vi "SWERVE_DRIVE_DASH_WRITE.vi"   [LabVIEW 2023]
uses:
  SWERVE_DRIVE_GLOBALS.vi
  <vilib>/Rock Robotics/Network Tables/NT Write Numeric Array.vi
  <vilib>/Rock Robotics/Network Tables/NT Write Boolean Array.vi
  <vilib>/Rock Robotics/Network Tables/NT Write Boolean.vi
  <vilib>/Rock Robotics/Network Tables/NT Write Number.vi
  <vilib>/Rock Robotics/WPI/ThirdParty/JAS_Junk/TrajLib/Trajectory_Library.lvlib
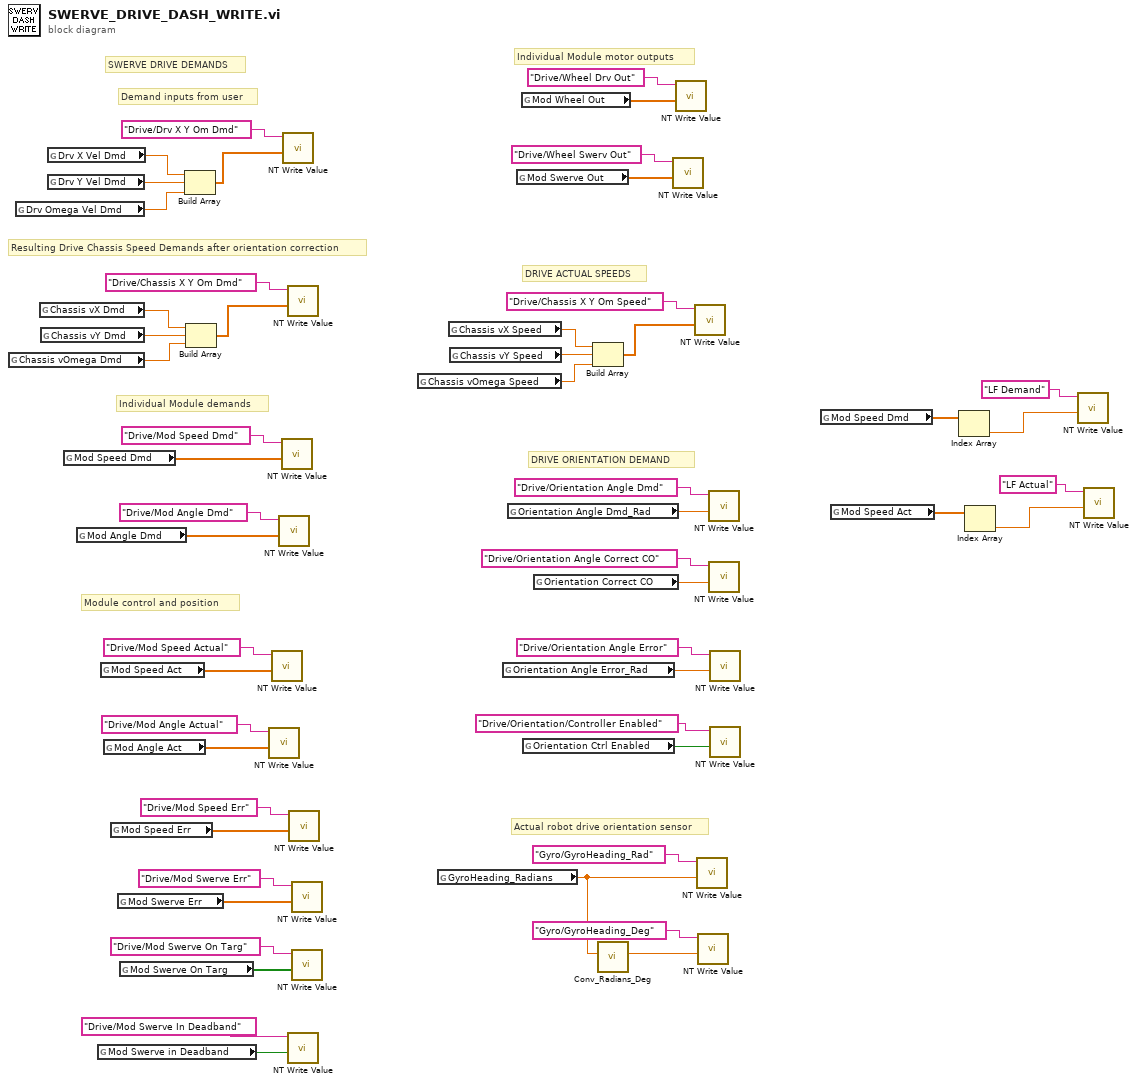
[diagram p0: block diagram]
diagram:
  # "Module control and position"
  # "Actual robot drive orientation sensor"
  # "DRIVE ACTUAL SPEEDS"
  # "DRIVE ORIENTATION DEMAND"
  # "Individual Module motor outputs"
  # "Individual Module demands"
  # "Resulting Drive Chassis Speed Demands after orientation correction"
  # "Demand inputs from user"
  # "SWERVE DRIVE DEMANDS"
  n1 = global read "SWERVE_DRIVE_GLOBALS.vi" "Chassis vOmega Dmd"() -> (w28:dbl)
  n2 = global read "SWERVE_DRIVE_GLOBALS.vi" "Drv Omega Vel Dmd"() -> (w31:dbl)
  n3 = global read "SWERVE_DRIVE_GLOBALS.vi" "Chassis vX Dmd"() -> (w30:dbl)
  n4 = global read "SWERVE_DRIVE_GLOBALS.vi" "Chassis vY Dmd"() -> (w29:dbl)
  n5 = global read "SWERVE_DRIVE_GLOBALS.vi" "Drv X Vel Dmd"() -> (w33:dbl)
  n6 = global read "SWERVE_DRIVE_GLOBALS.vi" "Drv Y Vel Dmd"() -> (w32:dbl)
  n7 = global read "SWERVE_DRIVE_GLOBALS.vi" "Mod Speed Dmd"() -> (w27:dbl[])
  n8 = global read "SWERVE_DRIVE_GLOBALS.vi" "Mod Angle Dmd"() -> (w26:dbl[])
  n9 = global read "SWERVE_DRIVE_GLOBALS.vi" "Mod Swerve in Deadband"() -> (w21:bool)
  n10 = global read "SWERVE_DRIVE_GLOBALS.vi" "Mod Speed Act"() -> (w25:dbl[])
  n11 = global read "SWERVE_DRIVE_GLOBALS.vi" "Mod Angle Act"() -> (w24:dbl[])
  n12 = global read "SWERVE_DRIVE_GLOBALS.vi" "Mod Speed Err"() -> (w23:dbl[])
  n13 = global read "SWERVE_DRIVE_GLOBALS.vi" "Mod Swerve Err"() -> (w22:dbl[])
  n14 = global read "SWERVE_DRIVE_GLOBALS.vi" "Mod Swerve On Targ"() -> (w20:bool[])
  n15 = Build Array(w33, w32, w31) -> (w37:dbl[])
  n16 = Build Array(w30, w29, w28) -> (w39:dbl[])
  n17 = call-poly <vilib>:"NT Write Value.vi"("value"=w24, "name"="Drive/Mod Angle Actual" ("Name")) -> ()  [unwired: 9 in, 1 out]
  n18 = call-poly <vilib>:"NT Write Value.vi"("value"=w25, "name"="Drive/Mod Speed Actual" ("Name")) -> ()  [unwired: 9 in, 1 out]
  n19 = call-poly <vilib>:"NT Write Value.vi"("value"=w26, "name"="Drive/Mod Angle Dmd" ("Name")) -> ()  [unwired: 9 in, 1 out]
  n20 = call-poly <vilib>:"NT Write Value.vi"("value"=w27, "name"="Drive/Mod Speed Dmd" ("Name")) -> ()  [unwired: 9 in, 1 out]
  n21 = call-poly <vilib>:"NT Write Value.vi"("value"=w37, "name"="Drive/Drv X Y Om Dmd" ("Name")) -> ()  [unwired: 9 in, 1 out]
  n22 = call-poly <vilib>:"NT Write Value.vi"("value"=w39, "name"="Drive/Chassis X Y Om Dmd" ("Name")) -> ()  [unwired: 9 in, 1 out]
  n23 = call-poly <vilib>:"NT Write Value.vi"("value"=w21, "name"="Drive/Mod Swerve In Deadband" ("Name")) -> ()  [unwired: 9 in, 1 out]
  n24 = call-poly <vilib>:"NT Write Value.vi"("value"=w23, "name"="Drive/Mod Speed Err" ("Name")) -> ()  [unwired: 9 in, 1 out]
  n25 = call-poly <vilib>:"NT Write Value.vi"("value"=w22, "name"="Drive/Mod Swerve Err" ("Name")) -> ()  [unwired: 9 in, 1 out]
  n26 = call-poly <vilib>:"NT Write Value.vi"("value"=w20, "name"="Drive/Mod Swerve On Targ" ("Name")) -> ()  [unwired: 9 in, 1 out]
  n27 = global read "SWERVE_DRIVE_GLOBALS.vi" "Chassis vOmega Speed"() -> (w9:dbl)
  n28 = global read "SWERVE_DRIVE_GLOBALS.vi" "GyroHeading_Radians"() -> (w12:dbl)
  n29 = global read "SWERVE_DRIVE_GLOBALS.vi" "Chassis vX Speed"() -> (w11:dbl)
  n30 = global read "SWERVE_DRIVE_GLOBALS.vi" "Chassis vY Speed"() -> (w10:dbl)
  n31 = global read "SWERVE_DRIVE_GLOBALS.vi" "Orientation Angle Error_Rad"() -> (w15:dbl)
  n32 = global read "SWERVE_DRIVE_GLOBALS.vi" "Orientation Angle Dmd_Rad"() -> (w17:dbl)
  n33 = global read "SWERVE_DRIVE_GLOBALS.vi" "Mod Swerve Out"() -> (w19:dbl[])
  n34 = global read "SWERVE_DRIVE_GLOBALS.vi" "Mod Wheel Out"() -> (w18:dbl[])
  n35 = global read "SWERVE_DRIVE_GLOBALS.vi" "Orientation Ctrl Enabled"() -> (w2:bool)
  n36 = global read "SWERVE_DRIVE_GLOBALS.vi" "Orientation Correct CO"() -> (w16:dbl)
  n37 = Build Array(w11, w10, w9) -> (w47:dbl[])
  n38 = call <vilib>:"Conv_Radians_Deg.vi"("Radians"=w12) -> ("Degrees"=w13:dbl)  [unwired: 10 in]
  n39 = call-poly <vilib>:"NT Write Value.vi"("value"=w19, "name"="Drive/Wheel Swerv Out" ("Name")) -> ()  [unwired: 9 in, 1 out]
  n40 = call-poly <vilib>:"NT Write Value.vi"("value"=w18, "name"="Drive/Wheel Drv Out" ("Name")) -> ()  [unwired: 9 in, 1 out]
  n41 = call-poly <vilib>:"NT Write Value.vi"("value"=w47, "name"="Drive/Chassis X Y Om Speed" ("Name")) -> ()  [unwired: 9 in, 1 out]
  n42 = call-poly <vilib>:"NT Write Value.vi"("value"=w12, "name"="Gyro/GyroHeading_Rad" ("Name")) -> ()  [unwired: 9 in, 1 out]
  n43 = call-poly <vilib>:"NT Write Value.vi"("value"=w13, "name"="Gyro/GyroHeading_Deg" ("Name")) -> ()  [unwired: 9 in, 1 out]
  n44 = call-poly <vilib>:"NT Write Value.vi"("value"=w17, "name"="Drive/Orientation Angle Dmd" ("Name")) -> ()  [unwired: 9 in, 1 out]
  n45 = call-poly <vilib>:"NT Write Value.vi"("value"=w16, "name"="Drive/Orientation Angle Correct CO" ("Name")) -> ()  [unwired: 9 in, 1 out]
  n46 = call-poly <vilib>:"NT Write Value.vi"("value"=w15, "name"="Drive/Orientation Angle Error" ("Name")) -> ()  [unwired: 9 in, 1 out]
  n47 = call-poly <vilib>:"NT Write Value.vi"("value"=w2, "name"="Drive/Orientation/Controller Enabled" ("Name")) -> ()  [unwired: 9 in, 1 out]
  n48 = global read "SWERVE_DRIVE_GLOBALS.vi" "Mod Speed Dmd"() -> (w8:dbl[])
  n49 = global read "SWERVE_DRIVE_GLOBALS.vi" "Mod Speed Act"() -> (w5:dbl[])
  n50 = Index Array(array=w8) -> (element=w6:dbl)  [unwired: 1 in]
  n51 = Index Array(array=w5) -> (element=w3:dbl)  [unwired: 1 in]
  n52 = call-poly <vilib>:"NT Write Value.vi"("value"=w6, "name"="LF Demand" ("Name")) -> ()  [unwired: 9 in, 1 out]
  n53 = call-poly <vilib>:"NT Write Value.vi"("value"=w3, "name"="LF Actual" ("Name")) -> ()  [unwired: 9 in, 1 out]
